vi "Protection.vi"(7 "RMS Value":dbl[](array[numeric]), 8 "10 Amps":dbl=400.0 format="%#_13g", 9 "Trigger 10 times":dbl, 10 "5 Amps":dbl=400.0 format="%#_13g", 11 "Trigger 2 times":dbl) -> (0 "Trigger":bool, 1 "Trigger 10 out":dbl, 3 "Trigger 2 out":dbl)   [LabVIEW 2022 SP3]
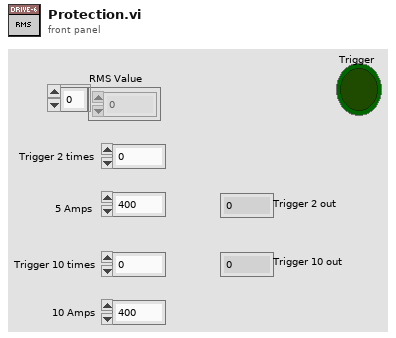
[diagram p1: front panel]
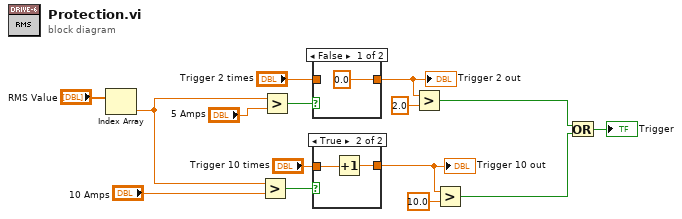
[diagram p0: block diagram]
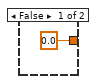
[diagram p2: hidden frame]
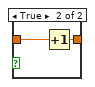
[diagram p3: hidden frame]
diagram:
  n1 = Index Array(array="RMS Value") -> (element=w6:dbl)  [unwired: 1 in]
  n2 = Greater?(x=w6, y="10 Amps") -> (0:w12:bool)
  n3 = Greater?(x=w6, y="5 Amps") -> (0:w8:bool)
  n4 = case shown="False" w8 {
    tunnel: "Trigger 2 times" -> [_ w18]
    tunnel: [0.0 w17] -> w4
    frame False {
    }
    frame True {
      n5 = Increment(x=w18) -> (x+1=w17:dbl)
    }
  }
  "Trigger 2 out" <- w4
  n6 = case shown="True" w12 {
    tunnel: "Trigger 10 times" -> [_ w21]
    tunnel: [0.0 w20] -> w9
    frame False {
    }
    frame True {
      n7 = Increment(x=w21) -> (x+1=w20:dbl)
    }
  }
  "Trigger 10 out" <- w9
  n8 = Greater?(x=w4, y=2.0) -> (0:w3:bool)
  n9 = Greater?(x=w9, y=10.0) -> (0:w2:bool)
  n10 = Or(x=w3, y=w2) -> (x .or. y?=→"Trigger":bool)
